vi "Push Token.vi"(7 "Type":T1, 8 "Error In":errorcluster, 9 "Content":string, 10 "Tag":string, 11 "Parser In":refnum<class "Parser.lvclass">) -> (0 "Error Out":errorcluster, 3 "Parser Out":refnum<class "Parser.lvclass">)   [LabVIEW 2017, in "Mustache.lvlib" / "Parser.lvclass"]
uses:
  Parser.lvclass
  Public/Controls/Token Types.ctl
  Parser.lvclass/Parser.ctl
  Public/Controls/Token.ctl
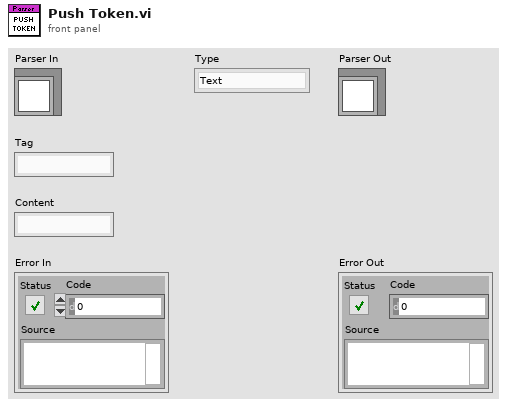
[diagram p1: front panel]
types:
  T1 = typedef "Mustache.lvlib/Parser.lvclass/Token Types.ctl" = enum16{"Text", "Escaped Tag", "Unescaped Tag", "Section", "Incomplete Section", "Partial"}
  T2 = typedef "Mustache.lvlib/Parser.lvclass/Token.ctl" = cluster{"Type":T1, "Data":variant}
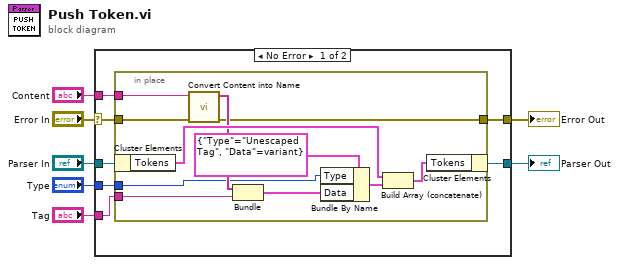
[diagram p0: block diagram]
diagram:
  n1 = case shown="No Error" "Error In" {
    selector: "Error In" -> [w8 w26]
    tunnel: "Tag" -> [w14 _]
    tunnel: [w13 w27] -> w6
    tunnel: [w12 w26] -> w5
    tunnel: "Parser In" -> [w11 w27]
    tunnel: "Content" -> [w10 _]
    tunnel: "Type" -> [w9 _]
    frame No Error {
      n2 = in-place {
        in-place-border: [w19] -> w12
        in-place-border: w8 -> [w18]
        in-place-border: w10 -> [w17]
        in-place-border: w14 -> [w16]
        in-place-border: w9 -> [w15]
        n3 = in-place-cluster #1(w11) -> ("Tokens"=w25:T2[])
        n4 = call "Convert Content into Name.vi"("Error In"=w18, "Content"=w17) -> ("Error Out"=w19:errorcluster, "Name"=w20:string[])  [unwired: 8 in]
        n5 = Bundle("Name"=w20, "Tag"=w16) -> (w21:cluster{"Name":string[], "Tag":string})  [unwired: 1 in]
        n6 = Bundle By Name(cluster=T2 {"Type"=enum."Unescaped Tag", "Data"=variant} ("Token"), "Type"=w15, "Data"=w21) -> (w22:T2)
        n7 = Build Array (concatenate)(w25, w22) -> (w24:T2[])
        n8 = in-place-cluster #1("Tokens"=w24) -> (w13:refnum<class "Parser.lvclass">)
      }
    }
    frame Error {
    }
  }
  "Parser Out" <- w6
  "Error Out" <- w5
